vi "PathPlanner_Trajectory_RecalculateValues.vi"(9 "Reversed":bool, 11 "PathPlannerStates":T1[](array[typedef]) {"HolonomicRotation"."SIN" format="%13.4f"; "HolonomicRotation"."COS" format="%13.4f"; "HolonomicRotation"."VALUE" format="%13.4f"; "AngularVelocity"."SIN" format="%13.4f"; "AngularVelocity"."COS" format="%13.4f"; "AngularVelocity"."VALUE" format="%13.4f"; "TrajectoryState"."POSE"."ROTATION"."SIN" format="%13.4f"; "TrajectoryState"."POSE"."ROTATION"."COS" format="%13.4f"; "TrajectoryState"."POSE"."ROTATION"."VALUE" format="%13.4f"; "TrajectoryState"."POSE"."TRANSLATION"."Y" format="%14.3f"; "TrajectoryState"."POSE"."TRANSLATION"."X" format="%14.3f"; "AngularAcceleration"."SIN" format="%13.4f"; "AngularAcceleration"."COS" format="%13.4f"; "AngularAcceleration"."VALUE" format="%13.4f"}) -> (3 "outPathPlannerStates":T1[](array[typedef]) {"HolonomicRotation"."SIN" format="%13.4f"; "HolonomicRotation"."COS" format="%13.4f"; "HolonomicRotation"."VALUE" format="%13.4f"; "AngularVelocity"."SIN" format="%13.4f"; "AngularVelocity"."COS" format="%13.4f"; "AngularVelocity"."VALUE" format="%13.4f"; "TrajectoryState"."POSE"."ROTATION"."SIN" format="%13.4f"; "TrajectoryState"."POSE"."ROTATION"."COS" format="%13.4f"; "TrajectoryState"."POSE"."ROTATION"."VALUE" format="%13.4f"; "TrajectoryState"."POSE"."TRANSLATION"."Y" format="%14.3f"; "TrajectoryState"."POSE"."TRANSLATION"."X" format="%14.3f"; "AngularAcceleration"."SIN" format="%13.4f"; "AngularAcceleration"."COS" format="%13.4f"; "AngularAcceleration"."VALUE" format="%13.4f"})   [LabVIEW 2019, in "PathPlanner.lvlib"]
uses:
  PathPlanner.lvlib
  PathPlannerState.ctl
  <vilib>/Rock Robotics/WPI/ThirdParty/JAS_Junk/TrajLib/ROTATION2D.ctl
  <vilib>/Rock Robotics/WPI/ThirdParty/JAS_Junk/TrajLib/TRAJ_STATE.ctl
  <vilib>/Rock Robotics/WPI/ThirdParty/JAS_Junk/TrajLib/POSE2D.ctl
  <vilib>/Rock Robotics/WPI/ThirdParty/JAS_Junk/TrajLib/TRANSLATION2D.ctl
  <vilib>/Rock Robotics/WPI/ThirdParty/JAS_Junk/TrajLib/Rotation_GetRadians.vi
  <vilib>/Rock Robotics/WPI/ThirdParty/JAS_Junk/TrajLib/Conv_Radians_Deg.vi
  <vilib>/Rock Robotics/WPI/ThirdParty/JAS_Junk/TrajLib/Conv_Deg_Radians.vi
  <vilib>/Rock Robotics/WPI/ThirdParty/JAS_Junk/TrajLib/Rotation_CreateAngle.vi
  <vilib>/Rock Robotics/WPI/ThirdParty/JAS_Junk/TrajLib/Rotation_UnaryMinus.vi
  <vilib>/Rock Robotics/WPI/ThirdParty/JAS_Junk/TrajLib/Rotation_RotateBy.vi
  <vilib>/Rock Robotics/WPI/ThirdParty/JAS_Junk/TrajLib/Rotation_CreateXY.vi
  <vilib>/Rock Robotics/WPI/ThirdParty/JAS_Junk/TrajLib/Util_CalcDist.vi
  <vilib>/Rock Robotics/WPI/ThirdParty/JAS_Junk/TrajLib/Trajectory_Library.lvlib
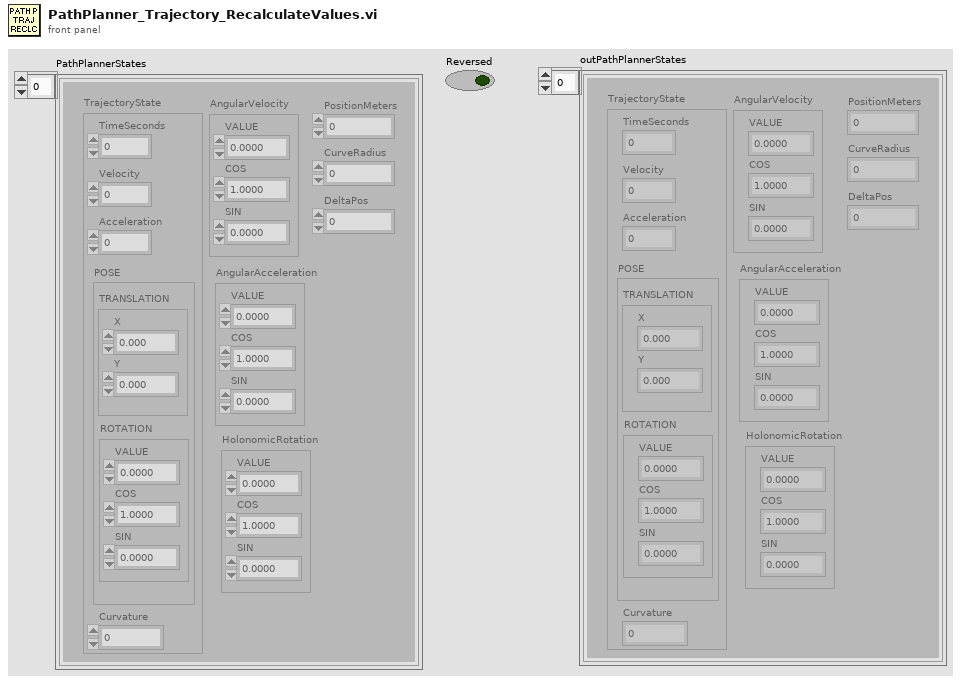
[diagram p1: front panel]
types:
  T1 = typedef "PathPlanner.lvlib/PathPlannerState.ctl" = cluster{"AngularAcceleration":T2, "PositionMeters":dbl, "TrajectoryState":T3, "AngularVelocity":T2, "HolonomicRotation":T2, "CurveRadius":dbl, "DeltaPos":dbl}
  T2 = typedef "Trajectory_Library.lvlib/ROTATION2D.ctl" = cluster{"VALUE":dbl, "COS":dbl, "SIN":dbl}
  T3 = typedef "Trajectory_Library.lvlib/TRAJ_STATE.ctl" = cluster{"TimeSeconds":dbl, "Velocity":dbl, "Acceleration":dbl, "POSE":T4, "Curvature":dbl}
  T4 = typedef "Trajectory_Library.lvlib/POSE2D.ctl" = cluster{"TRANSLATION":T5, "ROTATION":T2}
  T5 = typedef "Trajectory_Library.lvlib/TRANSLATION2D.ctl" = cluster{"X":dbl, "Y":dbl}
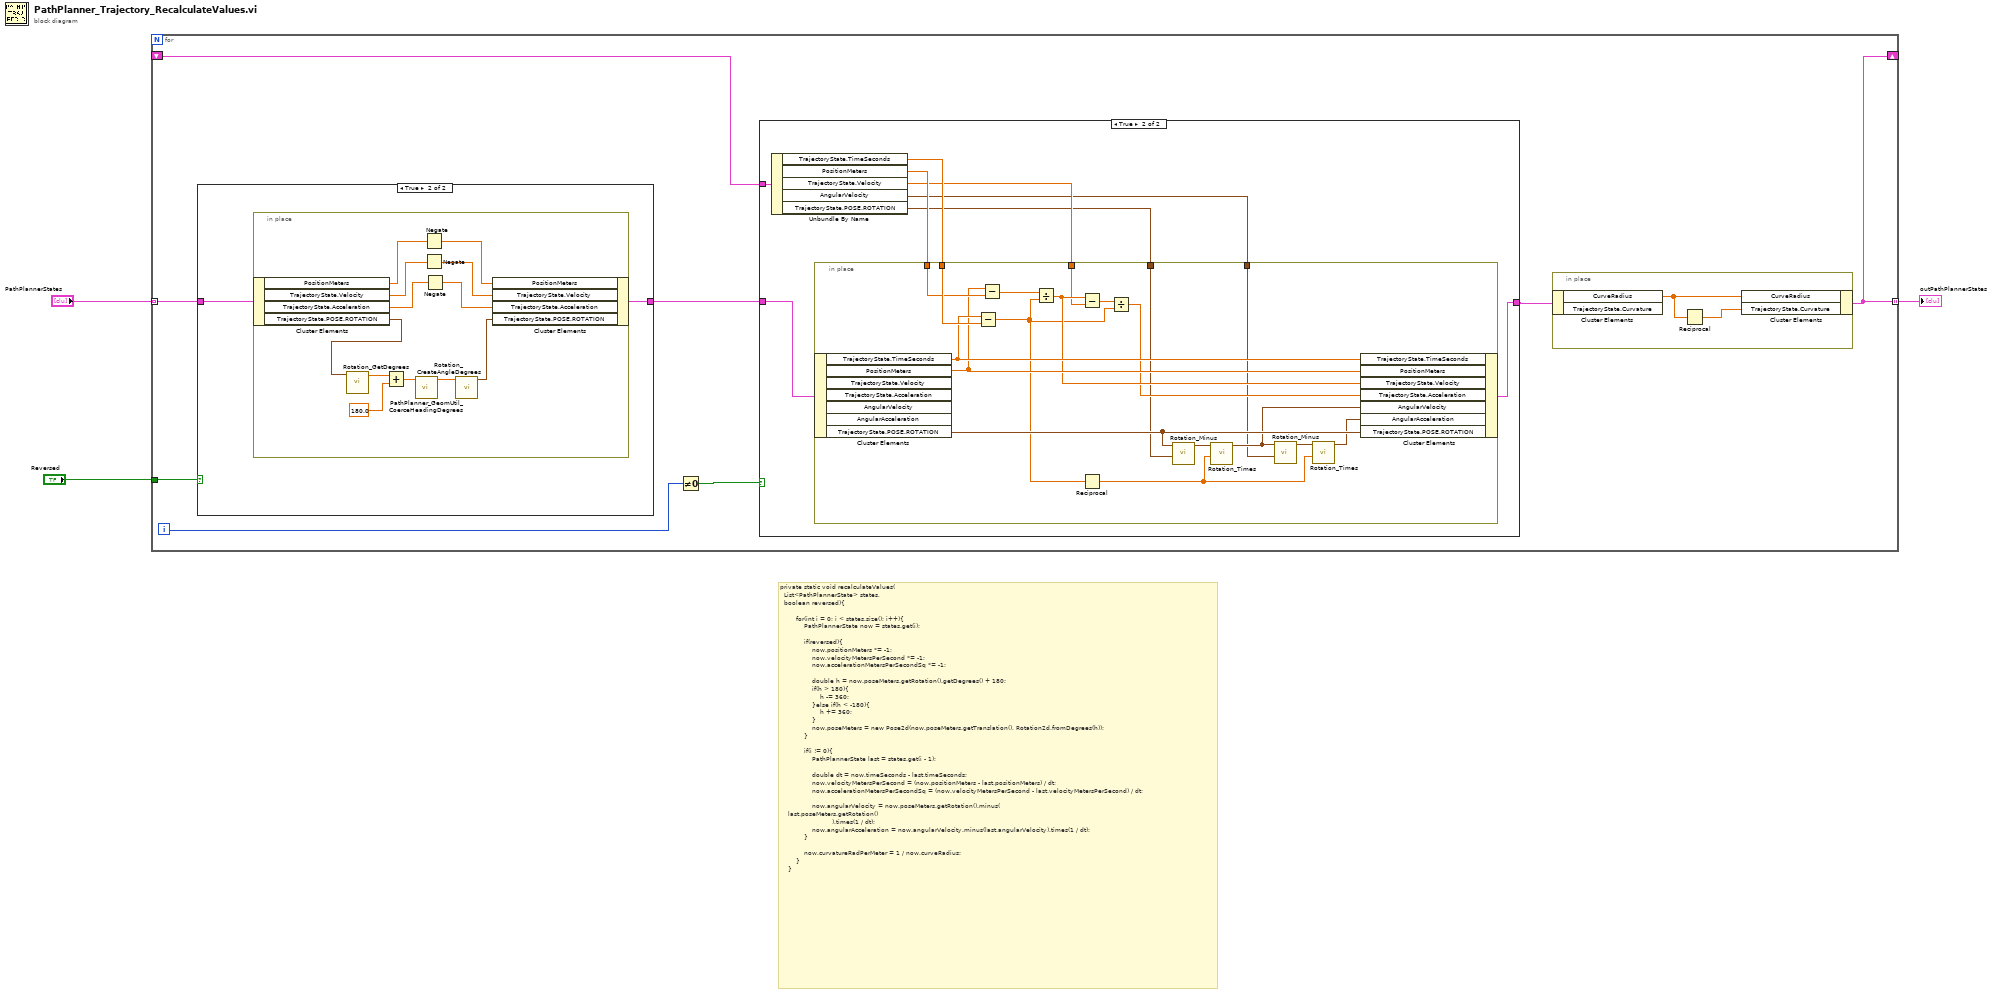
[diagram p0: block diagram]
diagram:
  # "private static void recalculateValues(\n\t\tList<PathPlannerState> states, \n\t\tboolean reversed){\n\n        for(int i = 0; i < states.size(); i++){\n            PathPlannerState now = states.get(i);\n\n            if(reversed){\n                now.positionMeters *= -1;\n                now.velocityMetersPerSecond *= -1;\n                now.accelerationMetersPerSecondSq *= -1;\n\n                double h = now.poseMeters.getRotation().getDegrees() + 180;\n                if(h > 180){\n                    h -= 360;\n                }else if(h < -180){\n                    h += 360;\n                }\n                now.poseMeters = new Pose2d(now.poseMeters.getTranslation(), Rotation2d.fromDegrees(h));\n            }\n\n            if(i != 0){\n                PathPlannerState last = states.get(i - 1);\n\n                double dt = now.timeSeconds - last.timeSeconds;\n                now.velocityMetersPerSecond = (now.positionMeters - last.positionMeters) / dt;\n                now.accelerationMetersPerSecondSq = (now.velocityMetersPerSecond - last.velocityMetersPerSecond) / dt;\n\n                now.angularVelocity = now.poseMeters.getRotation().minus(\n\t\t\t\tlast.poseMeters.getRotation()\n                          ).times(1 / dt);\n                now.angularAcceleration = now.angularVelocity.minus(last.angularVelocity).times(1 / dt);\n            }\n\n            now.curvatureRadPerMeter = 1 / now.curveRadius;\n        }\n    }"
  n1 = for {
    tunnel: "PathPlannerStates" -> [w10] mode=indexing
    tunnel: "Reversed" -> [w11]
    tunnel: [w4] -> w1 mode=indexing
    shift-right: [w4] -> _
    shift-left: _ -> [w6]
    i -> [w9]
    n2 = case shown="True" w11 {
      tunnel: w10 -> [w41 w43]
      tunnel: [w41 w42] -> w7
      frame False {
      }
      frame True {
        n3 = in-place {
          n4 = in-place-cluster #1(w43) -> ("PositionMeters"=w55:dbl, "TrajectoryState.Velocity"=w53:dbl, "TrajectoryState.Acceleration"=w51:dbl, "TrajectoryState.POSE.ROTATION"=w45:T2)
          n5 = call <vilib>:"Rotation_GetDegrees.vi"("in ROTATION"=w45) -> ("AngleDegrees"=w44:dbl)  [unwired: 10 in]
          n6 = Add(x=w44, y=180.0) -> (x+y=w46:dbl)
          n7 = call "PathPlanner_GeomUtil_CoerceHeadingDegrees.vi"("in Degrees"=w46) -> ("out Degrees"=w47:dbl)  [unwired: 10 in]
          n8 = Negate(x=w55) -> (-x=w54:dbl)
          n9 = Negate(x=w53) -> (-x=w52:dbl)
          n10 = Negate(x=w51) -> (-x=w50:dbl)
          n11 = call <vilib>:"Rotation_CreateAngleDegrees.vi"("Angle_Degrees"=w47) -> ("ROTATION"=w48:T2)  [unwired: 10 in]
          n12 = in-place-cluster #1("PositionMeters"=w54, "TrajectoryState.Velocity"=w52, "TrajectoryState.Acceleration"=w50, "TrajectoryState.POSE.ROTATION"=w48) -> (w42:T1)
        }
      }
    }
    n13 = Not Equal To 0?(x=w9) -> (x != 0?=w8:bool)
    n14 = case shown="True" w8 {
      tunnel: w7 -> [w14 w22]
      tunnel: [w14 w15] -> w5
      tunnel: w6 -> [_ w21]
      frame False {
      }
      frame True {
        n15 = Unbundle By Name(w21) -> ("TrajectoryState.TimeSeconds"=w20:dbl, "PositionMeters"=w19:dbl, "TrajectoryState.Velocity"=w18:dbl, "AngularVelocity"=w16:T2, "TrajectoryState.POSE.ROTATION"=w17:T2)
        n16 = in-place {
          in-place-border: w20 -> [w40]
          in-place-border: w19 -> [w39]
          in-place-border: w18 -> [w35]
          in-place-border: w17 -> [w30]
          in-place-border: w16 -> [w26]
          n17 = in-place-cluster #2(w22) -> ("TrajectoryState.TimeSeconds"=w38:dbl, "PositionMeters"=w37:dbl, "TrajectoryState.POSE.ROTATION"=w31:T2)  [unwired: 4 out]
          n18 = Subtract(x=w38, y=w40) -> (x-y=w24:dbl)
          n19 = Subtract(x=w37, y=w39) -> (x-y=w25:dbl)
          n20 = Divide(x=w25, y=w24) -> (x/y=w36:dbl)
          n21 = Subtract(x=w36, y=w35) -> (x-y=w34:dbl)
          n22 = Reciprocal(x=w24) -> (1/x=w23:dbl)
          n23 = Divide(x=w34, y=w24) -> (x/y=w33:dbl)
          n24 = call <vilib>:"Rotation_Minus.vi"("other ROTATION"=w30, "in ROTATION"=w31) -> ("out ROTATION"=w32:T2)  [unwired: 9 in]
          n25 = call <vilib>:"Rotation_Times.vi"("Scalar"=w23, "in ROTATION"=w32) -> ("out ROTATION"=w28:T2)  [unwired: 9 in]
          n26 = call <vilib>:"Rotation_Minus.vi"("other ROTATION"=w26, "in ROTATION"=w28) -> ("out ROTATION"=w29:T2)  [unwired: 9 in]
          n27 = call <vilib>:"Rotation_Times.vi"("Scalar"=w23, "in ROTATION"=w29) -> ("out ROTATION"=w27:T2)  [unwired: 9 in]
          n28 = in-place-cluster #2("TrajectoryState.TimeSeconds"=w38, "PositionMeters"=w37, "TrajectoryState.Velocity"=w36, "TrajectoryState.Acceleration"=w33, "AngularVelocity"=w28, "AngularAcceleration"=w27, "TrajectoryState.POSE.ROTATION"=w31) -> (w15:T1)
        }
      }
    }
    n29 = in-place {
      n30 = in-place-cluster #3(w5) -> ("CurveRadius"=w13:dbl)  [unwired: 1 out]
      n31 = Reciprocal(x=w13) -> (1/x=w12:dbl)
      n32 = in-place-cluster #3("CurveRadius"=w13, "TrajectoryState.Curvature"=w12) -> (w4:T1)
    }
  }
  "outPathPlannerStates" <- w1
